vi "User Interface.vi"(8 "error in":errorcluster, 11 "User Interface in":refnum<class "User Interface.lvclass">) -> (0 "error out":errorcluster, 3 "User Interface out":refnum<class "User Interface.lvclass">)   [LabVIEW 2020, in "RDMA.lvlib" / "RDMA Plugin User Interface.lvclass"]
uses:
  RDMA Plugin User Interface.lvclass
  DSF Core.lvlibp/Classes/User Interface/User Interface.lvclass
  Configuration/Plugin/RDMA Plugin Configuration.lvclass
  C:/git/fmussi-niveristand-data-sharing-framework-custom-device-plugins/Components/DSF Core.lvlibp/Classes/Configuration/Configuration.lvclass
panel:
  in  "Initialization Timeout [sec]":dbl
  # "RDMA Plugin Settings"
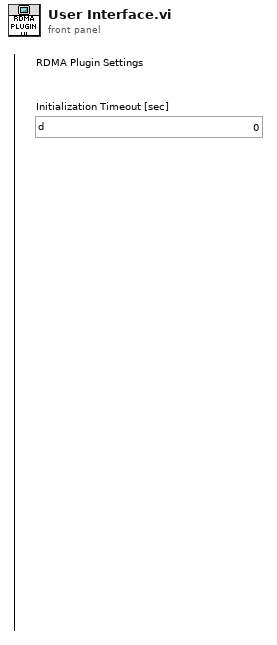
[diagram p1: front panel]
types:
  T1 = typedef "RDMA.lvlib/RDMA Plugin Configuration.lvclass/Plugin Settings.ctl" = cluster{"initialization timeout s":dbl}
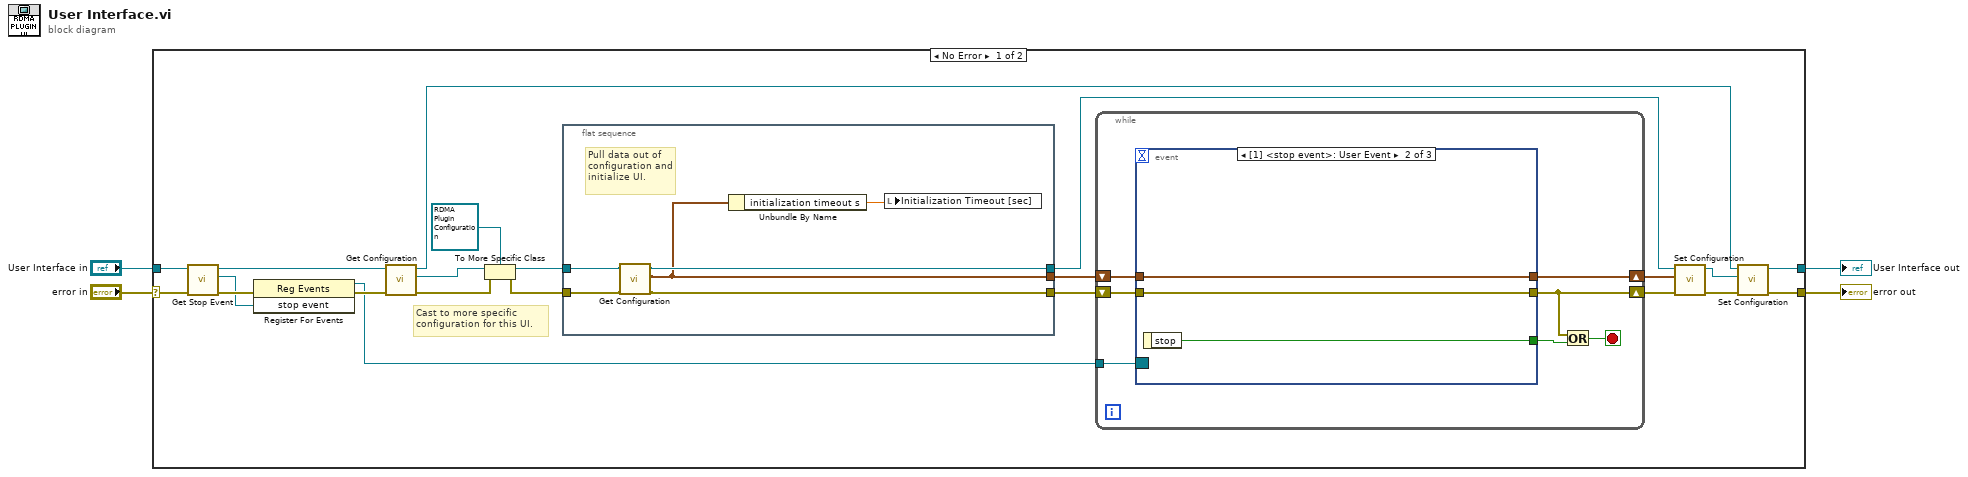
[diagram p0: block diagram]
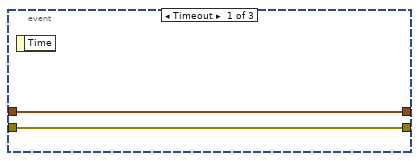
[diagram p2: hidden frame]
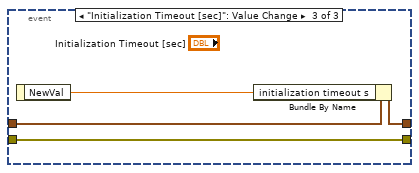
[diagram p3: hidden frame]
diagram:
  n1 = case shown="No Error" "error in" {
    selector: "error in" -> [w23 w50]
    tunnel: [w14 w50] -> w4
    tunnel: "User Interface in" -> [w22 w49]
    tunnel: [w13 w49] -> w1
    frame No Error {
      # "Cast to more specific configuration for this UI."
      n2 = call "Get Stop Event.vi"("error in (no error)"=w23, "User Interface in"=w22) -> ("error out"=w21:errorcluster, "stop event"=w20:refnum<user-event>, "User Interface out"=w19:refnum<class "User Interface.lvclass">)  [unwired: 7 in]
      n3 = register-events(error in=w21, w20) -> (reference out=w17:refnum<event-registration>, error out=w18:errorcluster)  [unwired: 1 in]
      n4 = call "Get Configuration.vi"("error in (no error)"=w18, "User Interface in"=w19) -> ("error out"=w16:errorcluster, "configuration"=w15:refnum<class "Configuration.lvclass">, "User Interface out"=w12:refnum<class "User Interface.lvclass">)  [unwired: 7 in]
      n5 = To More Specific Class(target class=refnum<class "RDMA Plugin Configuration.lvclass"> refnum ("RDMA.lvlib:RDMA Plugin Configuration.lvclass"), reference=w15, error in=w16) -> (specific class reference=w26:refnum<class "RDMA Plugin Configuration.lvclass">, error out=w24:errorcluster)
      n6 = flat-sequence {
        tunnel: [w30] -> w25
        tunnel: w24 -> [w31]
        tunnel: w26 -> [w32]
        tunnel: [w29] -> w7
        tunnel: [w28] -> w11
        frame #0 {
          # "Pull data out of configuration and initialize UI."
          n7 = call "Get Configuration.vi"("error in (no error)"=w31, "RDMA Plugin Configuration in"=w32) -> ("error out"=w30:errorcluster, "plugin settings"=w28:T1, "RDMA Plugin Configuration out"=w29:refnum<class "RDMA Plugin Configuration.lvclass">)  [unwired: 7 in]
          n8 = Unbundle By Name(w28) -> ("initialization timeout s"=w27:dbl)
          n9 = local write "Initialization Timeout [sec]"(w27) -> ()
        }
      }
      n10 = while {
        tunnel: w17 -> [w39]
        shift-right: [w37] -> w10
        shift-left: w25 -> [w38]
        shift-right: [w33] -> w8
        shift-left: w11 -> [w34]
        stop <- w36 stop-if-true
        n11 = event shown="[1] <stop event>: User Event" {
          selector: w39 -> [_ _ _]
          dyn-events: _ -> [_ _ _]
          timeout: _ -> [_ _ _]
          tunnel: [_ w43 _] -> w35
          tunnel: w38 -> [w41 w44 w48]
          tunnel: [w41 w44 w48] -> w37
          tunnel: w34 -> [w40 w42 w47]
          tunnel: [w40 w42 w46] -> w33
          event Timeout {
            n12 = event-data() -> ()  [unwired: 1 in, 1 out]
          }
          event User Event {
            n13 = event-data() -> ("stop"=w43:bool)  [unwired: 1 in]
          }
          event "Initialization Timeout [sec]": Value Change {
            n14 = event-data() -> ("NewVal"=w45:dbl)  [unwired: 1 in]
            n15 = Bundle By Name(cluster=w47, "initialization timeout s"=w45) -> (w46:T1)
          }
        }
        n16 = Or(x=w37, y=w35) -> (x .or. y?=w36:bool)
      }
      n17 = call "Set Configuration.vi"("error in (no error)"=w10, "plugin settings"=w8, "RDMA Plugin Configuration in"=w7) -> ("error out"=w9:errorcluster, "RDMA Plugin Configuration out"=w6:refnum<class "RDMA Plugin Configuration.lvclass">)  [unwired: 7 in]
      n18 = call "Set Configuration.vi"("error in (no error)"=w9, "configuration"=w6, "User Interface in"=w12) -> ("error out"=w14:errorcluster, "User Interface out"=w13:refnum<class "User Interface.lvclass">)  [unwired: 7 in]
    }
    frame Error {
    }
  }
  "error out" <- w4
  "User Interface out" <- w1
